vi "Configure VXI-11 Interface.vi"(8 "error in (no error)":errorcluster, 9 "Enable VXI-11 Interface (On)":bool=TRUE, 10 "Channel (1)":i32=1, 11 "VISA resource name":refnum<visa-resource-name>) -> (0 "error out":errorcluster, 3 "VISA resource name out":refnum<visa-resource-name>)   [LabVIEW 2015, in "Rohde&Schwarz CMXP Base.lvlib"]
doc: "Enables or disables the VXI-11 interface.\n\nAttribute:\nRSCMXPBASE_ATTR_ENABLE_VXI11_INTERFACE\n\nRemote-control command:\nSYSTem:COMMunicate:VXI<i>:GTR"
uses:
  <instrlib>/Rohde&Schwarz CMXP Base/Rohde&Schwarz CMXP Base.lvlib
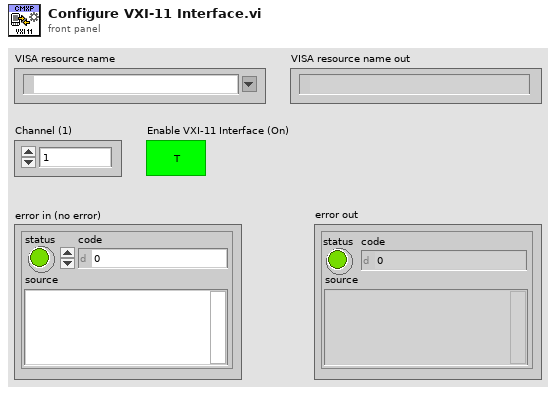
[diagram p1: front panel]
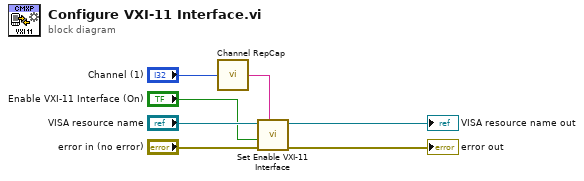
[diagram p0: block diagram]
diagram:
  n1 = call <instrlib>:"Channel RepCap.vi"("Channel In"="Channel (1)") -> ("Channel Out"=w2:string)  [unwired: 1 out]
  n2 = call "Set Enable VXI-11 Interface"("Repeated Capabilities"=w2, "error in (no error)"="error in (no error)", "Enable VXI-11 Interface (OFF)"="Enable VXI-11 Interface (On)", "instrument handle"="VISA resource name") -> ("error out"=→"error out":errorcluster, "instrument handle out"=→"VISA resource name out":refnum<visa-resource-name>)  [unwired: 6 in]
